vi "final cal x.vi"(0 "x0 base 1":dbl, 1 "x0 base 2":dbl, 2 "x0  base 3":dbl, 3 "d1":dbl, 4 "d2":dbl, 5 "d3":dbl) -> (16 "x":dbl)   [LabVIEW 2026]
uses:
  <vilib>/express/express arith-compare/Formula/XNode/ExpressFormulaBlockNode.xnode
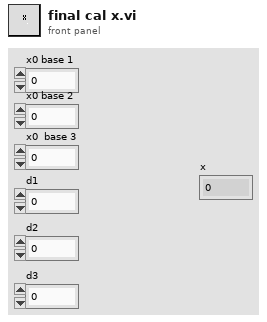
[diagram p1: front panel]
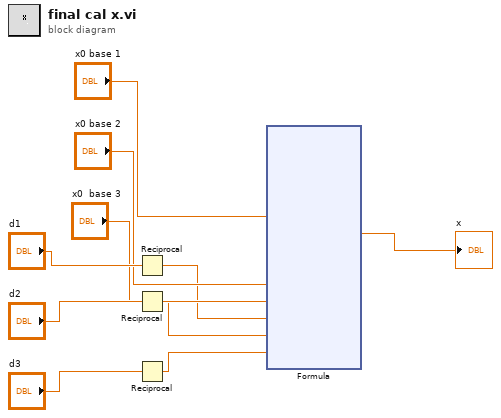
[diagram p0: block diagram]
diagram:
  n1 = Reciprocal(x="d1") -> (1/x=w4:dbl)
  n2 = Reciprocal(x="d2") -> (1/x=w3:dbl)
  n3 = Reciprocal(x="d3") -> (1/x=w2:dbl)
  n4 = xnode "Formula"("x1"="x0 base 1", "x2"="x0 base 2", "x3"="x0  base 3", "w1"=w4, "w2"=w3, "w3"=w2) -> ("Result"=→"x":dbl)  [unwired: 1 in, 1 out]
